vi "validate_configuration.vi"(8 "error in (no error)":errorcluster, 11 "configuration in":T1={"username"="", "password"="", "host"="", "type"=enum."ssh"}) -> (0 "error out":errorcluster, 3 "configuration out":T1={"username"="", "password"="", "host"="", "type"=enum."ssh"})   [LabVIEW 2015, in "lv-bin-plink.lvlib" / "v1.lvlib"]
uses:
  v1.lvlib
  _controls/configuration.ctl
  _controls/type.ctl
  _controls/error.ctl
  lv-bin-plink.lvlib
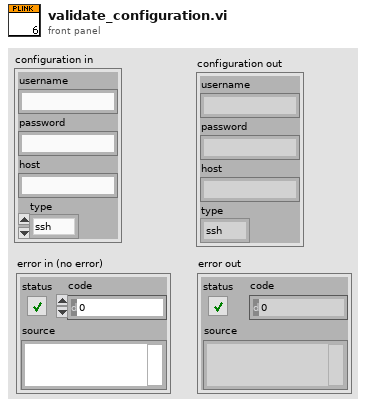
[diagram p1: front panel]
types:
  T1 = typedef "lv-bin-plink.lvlib/v1.lvlib/configuration.ctl" = cluster{"username":string, "password":string, "host":string, "type":T2}
  T2 = typedef "lv-bin-plink.lvlib/v1.lvlib/type.ctl" = enum16{"<type>", "ssh", "telnet", "rlogin", "raw", "serial"}
  T3 = typedef "lv-bin-plink.lvlib/error.ctl" = enum16{"<error>", "bad_configuration", "standard_error", "plink_x86_missing", "plink_x64_missing"}
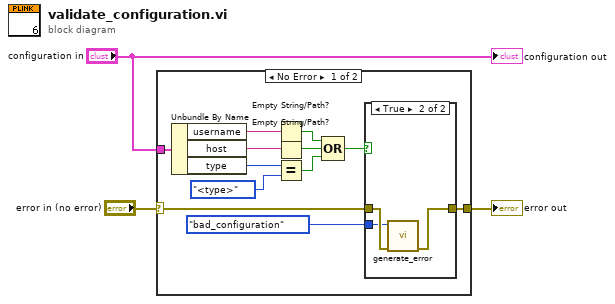
[diagram p0: block diagram]
diagram:
  n1 = case shown="No Error" "error in (no error)" {
    selector: "error in (no error)" -> [w7 w20]
    tunnel: "configuration in" -> [w15 _]
    tunnel: [w5 w20] -> w1
    frame No Error {
      n2 = Unbundle By Name(w15) -> ("username"=w14:string, "host"=w13:string, "type"=w12:T2)
      n3 = Empty String/Path?(string/path=w14) -> (empty?=w11:bool)
      n4 = Empty String/Path?(string/path=w13) -> (empty?=w10:bool)
      n5 = Equal?(x=w12, y=type."<type>" ("type")) -> (x = y?=w9:bool)
      n6 = Compound Arithmetic op=OR(w11, w10, w9) -> (w6:bool)
      n7 = case shown="True" w6 {
        tunnel: w7 -> [w16 w19]
        tunnel: [w16 w18] -> w5
        tunnel: error."bad_configuration" ("error") -> [_ w17]
        frame False {
        }
        frame True {
          n8 = call "generate_error.vi"("error in (no error)"=w19, "error"=w17) -> ("error out"=w18:errorcluster)  [unwired: 9 in]
        }
      }
    }
    frame Error {
    }
  }
  "error out" <- w1
  "configuration out" <- "configuration in"
